vi "Process PDC Configuration.vi"(7 "Pseudo PDC ID":i32, 8 "error in (no error)":errorcluster, 10 "PDC Configuration":T1, 11 "Phasor Data Concentrator in":refnum<class "Phasor Data Concentrator.lvclass">) -> (0 "error out":errorcluster, 3 "Phasor Data Concentrator out":refnum<class "Phasor Data Concentrator.lvclass">)   [LabVIEW 2018, in "S3DK.lvlib" / "PMU Recorder Light.lvlib" / "Phasor Data Concentrator.lvclass"]
uses:
  Phasor Data Concentrator.lvclass
  Phasor Data Concentrator.lvclass/Phasor Data Concentrator.ctl
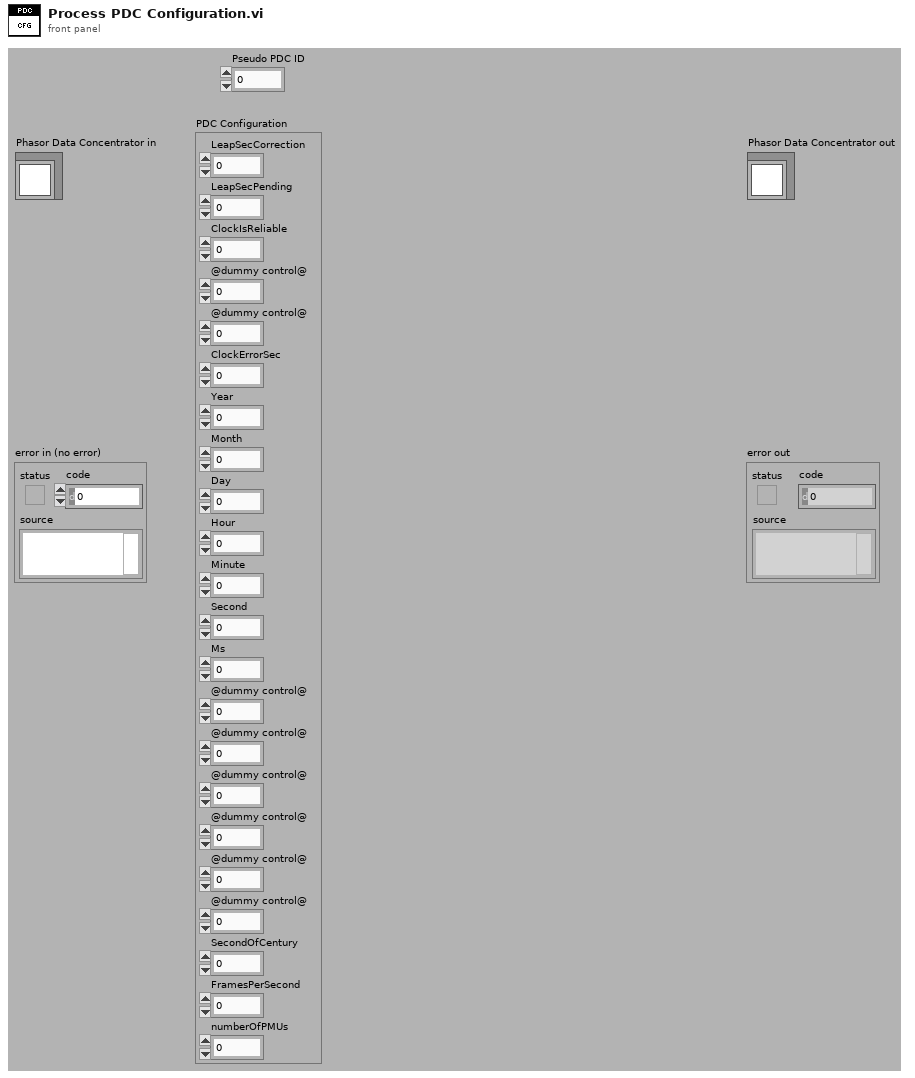
[diagram p1: front panel]
types:
  T1 = cluster{"LeapSecCorrection":i32, "LeapSecPending":u8, "ClockIsReliable":u8, "@dummy control@":i8, "@dummy control@":i8, "ClockErrorSec":sgl, "Year":i16, "Month":i16, "Day":i16, "Hour":i16, "Minute":i16, "Second":i16, "Ms":i16, "@dummy control@":i8, "@dummy control@":i8, "@dummy control@":i8, "@dummy control@":i8, "@dummy control@":i8, "@dummy control@":i8, "SecondOfCentury":dbl, "FramesPerSecond":sgl, "numberOfPMUs":i32}
  T2 = cluster{"Pseudo PDC ID":i32, "Leap Sec Correction":i32, "Leap Sec Pending":u8, "Clock Is Reliable":u8, "Clock Error Sec":sgl, "Frames Per Second":sgl, "Number Of PMUs":i32}
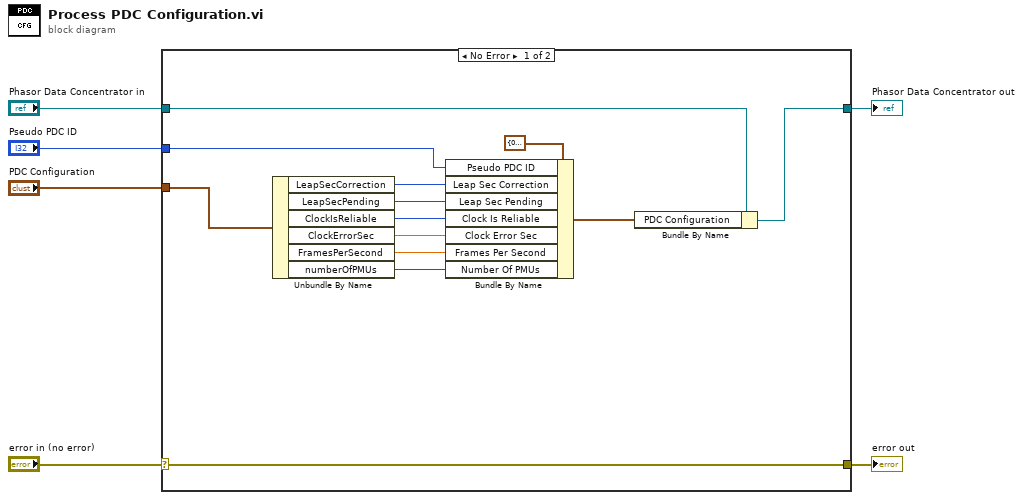
[diagram p0: block diagram]
diagram:
  n1 = case shown="No Error" "error in (no error)" {
    selector: "error in (no error)" -> [w19 w21]
    tunnel: [w19 w21] -> w5
    tunnel: [w17 w20] -> w3
    tunnel: "Phasor Data Concentrator in" -> [w18 w20]
    tunnel: "PDC Configuration" -> [w16 _]
    tunnel: "Pseudo PDC ID" -> [w14 _]
    frame No Error {
      n2 = Unbundle By Name(w16) -> ("LeapSecCorrection"=w13:i32, "LeapSecPending"=w12:u8, "ClockIsReliable"=w11:u8, "ClockErrorSec"=w10:sgl, "FramesPerSecond"=w9:sgl, "numberOfPMUs"=w8:i32)
      n3 = Bundle By Name(cluster=T2 {"Pseudo PDC ID"=0, "Leap Sec Correction"=0, "Leap Sec Pending"=0, "Clock Is Reliable"=0, "Clock Error Sec"=0.0, "Frames Per Second"=0.0, "Number Of PMUs"=0} ("PDC Configuration"), "Pseudo PDC ID"=w14, "Leap Sec Correction"=w13, "Leap Sec Pending"=w12, "Clock Is Reliable"=w11, "Clock Error Sec"=w10, "Frames Per Second"=w9, "Number Of PMUs"=w8) -> (w7:T2)
      n4 = Bundle By Name(cluster=w18, "PDC Configuration"=w7) -> (w17:refnum<class "Phasor Data Concentrator.lvclass">)
    }
    frame Error {
    }
  }
  "error out" <- w5
  "Phasor Data Concentrator out" <- w3
